vi "Wait phase sensor double.vi"(4 "Phase sensor number 2":i32, 5 "Phase sensor number 1":i32, 6 "Sense 2 T/F":bool=TRUE, 7 "Sense 1 T/F":bool=TRUE, 8 "error in (no error)":errorcluster, 11 "Sensitivity time (ms)":u32) -> (0 "error IO":errorcluster)   [LabVIEW 2017]
panel:
  out "Signal 2":bool
  out "Stop":bool
  out "Signal 1":bool
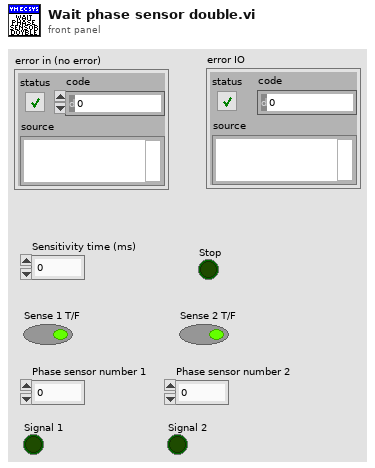
[diagram p1: front panel]
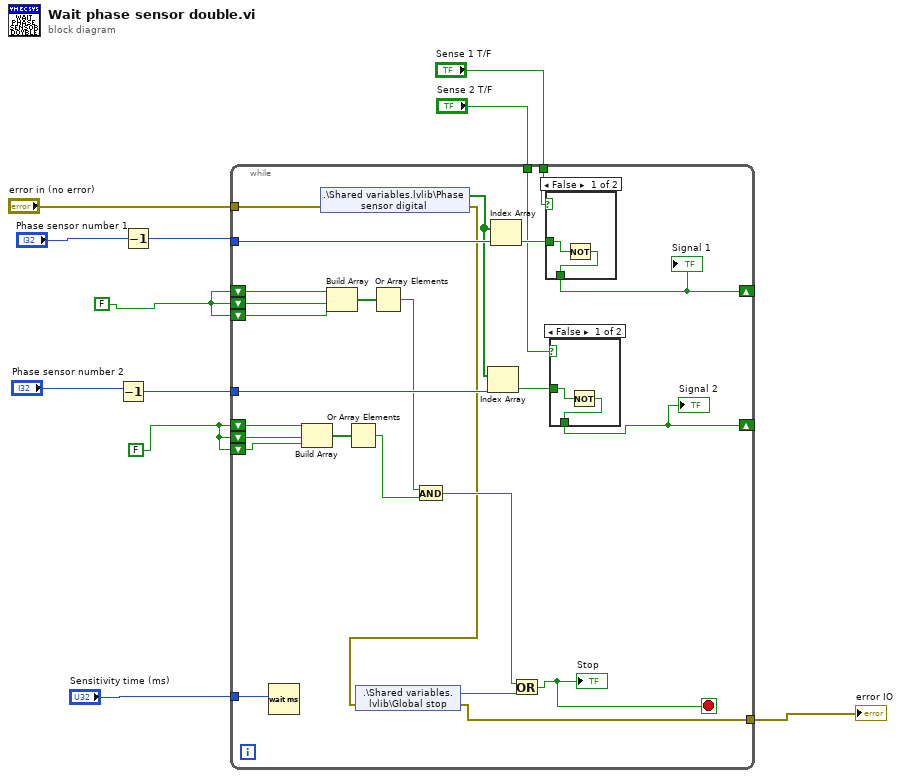
[diagram p0: block diagram]
diagram:
  w2 = FALSE ("Boolean")
  w7 = FALSE ("Boolean")
  n1 = Decrement(x="Phase sensor number 2") -> (x-1=w4:i32)
  n2 = Decrement(x="Phase sensor number 1") -> (x-1=w11:i32)
  n3 = while {
    shift-right: [w28] -> _
    shift-left: w7 -> [w37]
    shift-left: w7 -> [w36]
    shift-left: w7 -> [w35]
    tunnel: w11 -> [w33]
    tunnel: "Sensitivity time (ms)" -> [w32]
    tunnel: "error in (no error)" -> [w31]
    tunnel: "Sense 1 T/F" -> [w30]
    tunnel: w4 -> [w26]
    tunnel: "Sense 2 T/F" -> [w25]
    shift-right: [w23] -> _
    shift-left: w2 -> [w21]
    shift-left: w2 -> [w20]
    shift-left: w2 -> [w19]
    tunnel: [w12] -> w1
    stop <- w14 stop-if-true
    n4 = Wait (ms)(milliseconds to wait=w32) -> ()  [unwired: 1 out]
    n5 = Build Array(w21, w20, w19) -> (w22:bool[])
    n6 = shared-variable ".\\Shared variables.lvlib\\Phase sensor digital"(error in=w31) -> (w27:bool[], error out=w13:errorcluster)
    n7 = Build Array(w37, w36, w35) -> (w34:bool[])
    n8 = Or Array Elements(Boolean array=w22) -> (logical OR=w17:bool)
    n9 = shared-variable ".\\Shared variables.lvlib\\Global stop"(error in=w13) -> (w15:bool, error out=w12:errorcluster)
    n10 = Or Array Elements(Boolean array=w34) -> (logical OR=w18:bool)
    n11 = And(x=w18, y=w17) -> (x .and. y?=w16:bool)
    n12 = Index Array(array=w27, index=w26) -> (element=w24:bool)
    n13 = Index Array(array=w27, index=w33) -> (element=w29:bool)
    n14 = Or(x=w16, y=w15) -> (x .or. y?=w14:bool)
    "Stop" <- w14
    n15 = case shown="False" w30 {
      tunnel: w29 -> [w42 w43]
      tunnel: [w41 w43] -> w28
      frame False {
        n16 = Not(x=w42) -> (.not. x?=w41:bool)
      }
      frame True {
      }
    }
    "Signal 1" <- w28
    n17 = case shown="False" w25 {
      tunnel: w24 -> [w39 w40]
      tunnel: [w38 w40] -> w23
      frame False {
        n18 = Not(x=w39) -> (.not. x?=w38:bool)
      }
      frame True {
      }
    }
    "Signal 2" <- w23
  }
  "error IO" <- w1
